vi "Main.vi"() -> ()   [LabVIEW 2017]
doc: "The myRIO Project template acquires acceleration data from the onboard accelerometer and displays the changes of acceleration values in a waveform chart."
uses:
  <vilib>/myRIO/Instrument Drivers/Onboard IO/I2C/typedefs/I2C User Configuration.ctl
  <vilib>/myRIO/Instrument Drivers/Onboard IO/I2C/typedefs/I2C Transfer Rate.ctl
  <vilib>/myRIO/Instrument Drivers/Onboard IO/I2C/typedefs/I2C Reference.ctl
  <vilib>/myRIO/Common/Instrument Driver Framework/Utilities/typedefs/myRIO Generic Hardware Reference.ctl
  <vilib>/myRIO/Common/Instrument Driver Framework/Utilities/typedefs/Hardware Version Enum.ctl
  <vilib>/myRIO/Common/Instrument Driver Framework/Utilities/typedefs/myRIO v1.0 Reference.ctl
  <vilib>/myRIO/Common/Instrument Driver Framework/Utilities/typedefs/Generic FPGA Reference.ctl
  <vilib>/myRIO/Common/Instrument Driver Framework/myRIO v1.0/I2C/typedefs/I2C Channels Enum.ctl
  <vilib>/myRIO/Instrument Drivers/Onboard IO/I2C/typedefs/I2C Configuration.ctl
  <vilib>/userdefined/High Color/nirio_resource_hc.ctl
  <vilib>/myRIO/Common/Instrument Driver Framework/myRIO v1.0/I2C/vis/myRIO v1.1 Open I2C.vi
  <vilib>/myRIO/Common/Instrument Driver Framework/Utilities/vis/Validate Channels.vi
  <vilib>/myRIO/Common/Instrument Driver Framework/myRIO v1.0/I2C/vis/myRIO v1.0 Reserve I2C.vi
  <vilib>/myRIO/Common/Instrument Driver Framework/myRIO v1.0/UART/vis/myRIO v1.0 Close UART.vi
  <vilib>/myRIO/Common/Instrument Driver Framework/myRIO v1.0/I2C/vis/myRIO v1.0 Build MUX Configuration I2C.vi
  <vilib>/myRIO/Common/Instrument Driver Framework/myRIO v1.0/Resource Manager/vis/myRIO v1.0 Reserve Channel List.vi
  <vilib>/myRIO/Common/Instrument Driver Framework/myRIO v1.0/Resource Manager/vis/myRIO v1.0 Create Configuration List.vi
  <vilib>/myRIO/Common/Instrument Driver Framework/myRIO v1.0/Resource Manager/vis/myRIO v1.0 Reserve Channel.vi
  <vilib>/myRIO/Common/Instrument Driver Framework/myRIO v1.0/Resource Manager/vis/myRIO v1.0 Unreserve Channel.vi
  <vilib>/myRIO/Common/Instrument Driver Framework/myRIO v1.0/Resource Manager/vis/myRIO v1.0 Build Mutex Name.vi
  <vilib>/Utility/VariantDataType/GetNumericInfo.vi
  <vilib>/Utility/error.llb/Error Cluster From Error Code.vi
  <vilib>/myRIO/Common/Instrument Driver Framework/myRIO v1.0/myRIO v1.1 Open.vi
  <vilib>/myRIO/Common/Instrument Driver Framework/Utilities/vis/IO Manager.vi
  <vilib>/myRIO/Common/Instrument Driver Framework/Utilities/vis/Configuration Manager.vi
  <vilib>/myRIO/Common/Instrument Driver Framework/myRIO v1.0/Resource Manager/vis/myRIO v1.0 Configure IO.vi
  <vilib>/myRIO/Common/Instrument Driver Framework/myRIO v1.0/myRIO v1.0 Close.vi
  <vilib>/myRIO/Common/Instrument Driver Framework/myRIO v1.0/I2C/vis/myRIO v1.0 Configure I2C.vi
  <vilib>/myRIO/Common/Instrument Driver Framework/myRIO v1.0/I2C/vis/myRIO v1.0 Write I2C.vi
  <vilib>/myRIO/Common/Instrument Driver Framework/myRIO v1.0/I2C/vis/myRIO v1.0 Read I2C.vi
  <vilib>/myRIO/Common/Instrument Driver Framework/Utilities/vis/FPGA Ref Manager.vi
  <vilib>/myRIO/Common/Instrument Driver Framework/myRIO v1.0/myRIO v1.0 Reset FPGA.vi
  <vilib>/myRIO/Common/Instrument Driver Framework/myRIO v1.0/IRQ/vis/myRIO v1.0 IRQ Info FGV.vi
  <vilib>/myRIO/Common/Instrument Driver Framework/myRIO v1.0/IRQ/vis/myRIO v1.0 Timer IRQ Info FGV.vi
  <vilib>/myRIO/Common/Instrument Driver Framework/myRIO v1.0/IRQ/vis/myRIO v1.0 ISR Agent.vi
  <vilib>/myRIO/Instrument Drivers/Onboard IO/I2C/vis/myRIO I2C Open.xnode
  <vilib>/myRIO/Instrument Drivers/Utilities/Utilities.lvlib
  <vilib>/myRIO/Instrument Drivers/Onboard IO/I2C/I2C.lvlib
  <vilib>/ptbypt/NI_PtbyPt.lvlib
panel:
  out "AC estimate (Vrms)":dbl format="%0.2f"
  out "DC estimate (V)":dbl format="%0.2f"
  out "l":u8
  out "h":u8
  out "Numeric Control":u16
  out "error out":errorcluster
  in  "Stop":bool
  # "Overview: The myRIO Project template acquires acceleration data from the onboard accelerometer and displays the changes of acceleration values in a waveform chart.\nInstructions:\n1. Check the myRIO target IP address in the project and make sure the target IP address is correct. \n2. Run this VI."
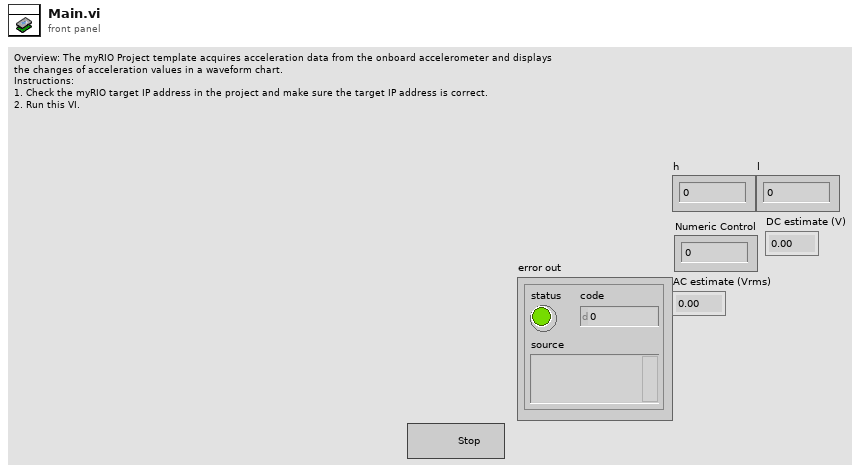
[diagram p1: front panel]
types:
  T1 = typedef "I2C.lvlib/I2C User Configuration.ctl" = cluster{"I2C Transfer Rate":T2}
  T2 = typedef "I2C.lvlib/I2C Transfer Rate.ctl" = enum16{"Standard mode (100 kbps)", "Fast mode (400 kbps)"}
  T3 = typedef "nirio_resource_hc.ctl" = tag
  T4 = typedef "Hardware Version Enum.ctl" = enum16{"Unknown", "myRIO-1900", "myRIO-1950", "roboRIO", "NI ELVIS RIO CM"}
  T5 = typedef "I2C.lvlib/I2C Reference.ctl" = cluster{"myRIO Reference":T6, "I2C Channels Enum":T9, "I2C Configuration":T10}
  T6 = typedef "myRIO Generic Hardware Reference.ctl" = cluster{"myRIO Model":T4, "myRIO Hardware Reference":T7}
  T7 = typedef "myRIO v1.0 Reference.ctl" = cluster{"Generic FPGA Reference":T8, "Allow multiple opens":bool}
  T8 = typedef "Generic FPGA Reference.ctl" = refnum<k20>
  T9 = typedef "I2C Channels Enum.ctl" = enum16{"Not Connected", "A/I2C", "B/I2C", "I2C/I2C"}
  T10 = typedef "I2C.lvlib/I2C Configuration.ctl" = cluster{"I2C Transfer Rate":T2}
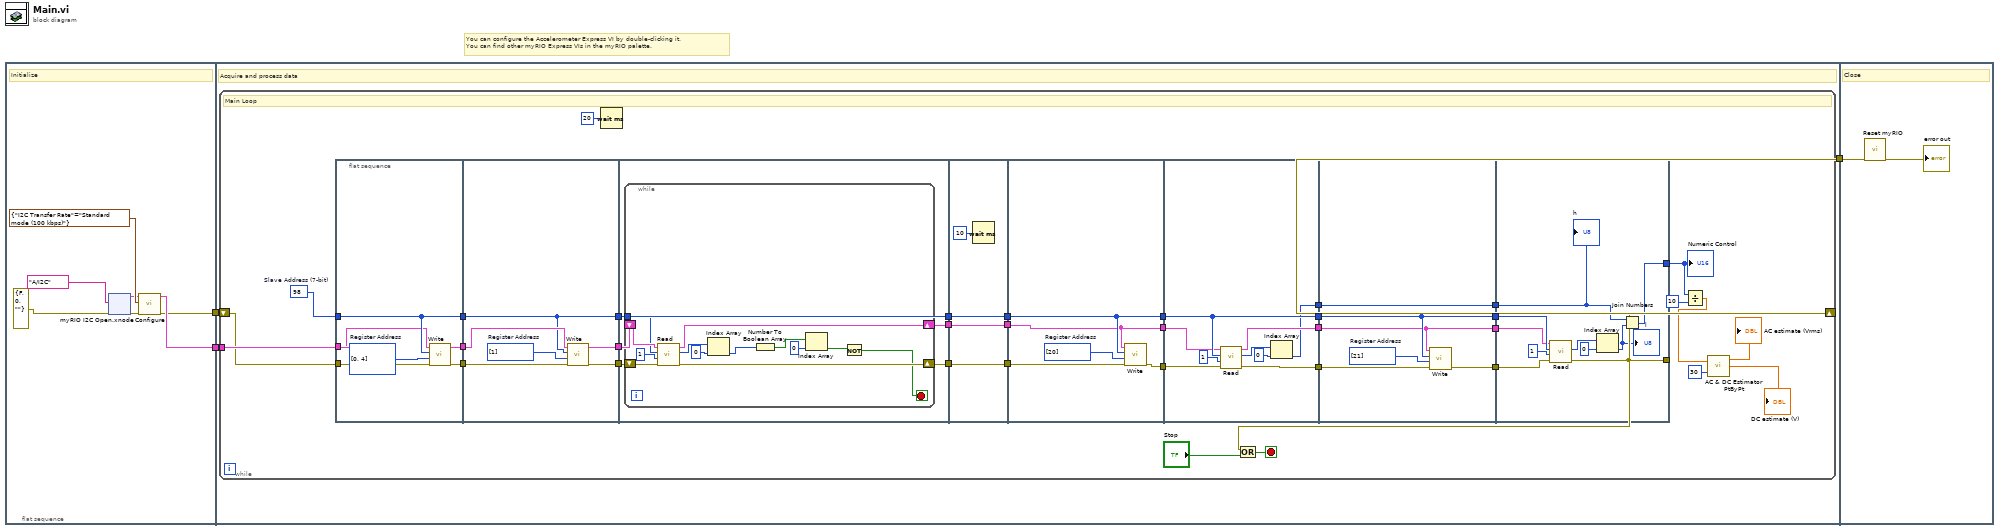
[diagram p0: block diagram]
diagram:
  # "You can configure the Accelerometer Express VI by double-clicking it.\nYou can find other myRIO Express VIs in the myRIO palette."
  n1 = flat-sequence {
    tunnel: [w5] -> w2
    tunnel: [w4] -> w1
    tunnel: [w28] -> w3
    tunnel: w2 -> [w27]
    tunnel: w1 -> [w29]
    tunnel: w3 -> [w131]
    frame #0 {
      # "Initialize"
      n2 = xnode "myRIO I2C Open.xnode"("error in (no error)"=errorcluster {"status"=FALSE, "code"=0, "source"=""}, "Channel Name"=tag "A/I2C") -> ("error out"=w7:errorcluster, "I2C Ref Out"=w8:T5)  [unwired: 1 in]
      n3 = call <vilib>:"Configure.vi"("error in (no error)"=w7, "I2C User Configuration"=T1 {"I2C Transfer Rate"=enum."Standard mode (100 kbps)"}, "I2C Ref In"=w8) -> ("error out"=w4:errorcluster, "I2C Ref Out"=w5:T5)  [unwired: 7 in]
    }
    frame #1 {
      # "Acquire and process data"
      n4 = while {
        shift-right: [w42] -> w28
        shift-left: w29 -> [w60]
        tunnel: w27 -> [w61]
        stop <- w64 stop-if-true
        w62 = u8 98  # Slave Address (7-bit)
        # "Main Loop"
        n5 = flat-sequence {
          tunnel: [w71] -> w59
          tunnel: [w70] -> w57
          tunnel: w62 -> [w68]
          tunnel: [w68] -> w55
          tunnel: w61 -> [w67]
          tunnel: w60 -> [w66]
          tunnel: w59 -> [w74]
          tunnel: [w73] -> w58
          tunnel: w57 -> [w75]
          tunnel: [w76] -> w56
          tunnel: w55 -> [w72]
          tunnel: [w72] -> w54
          tunnel: w58 -> [w82]
          tunnel: w56 -> [w81]
          tunnel: w54 -> [w78]
          tunnel: [w80] -> w41
          tunnel: [w79] -> w39
          tunnel: [w78] -> w37
          tunnel: w41 -> [w99]
          tunnel: [w99] -> w40
          tunnel: w39 -> [w98]
          tunnel: [w98] -> w38
          tunnel: w37 -> [w97]
          tunnel: [w97] -> w36
          tunnel: w40 -> [w100]
          tunnel: w38 -> [w103]
          tunnel: w36 -> [w101]
          tunnel: [w102] -> w53
          tunnel: [w101] -> w49
          tunnel: [w100] -> w45
          tunnel: w53 -> [w110]
          tunnel: [w109] -> w52
          tunnel: [w108] -> w50
          tunnel: w49 -> [w107]
          tunnel: [w107] -> w48
          tunnel: w45 -> [w106]
          tunnel: [w105] -> w44
          tunnel: w52 -> [w118]
          tunnel: [w117] -> w51
          tunnel: w50 -> [w115]
          tunnel: w48 -> [w116]
          tunnel: [w116] -> w47
          tunnel: [w115] -> w46
          tunnel: w44 -> [w114]
          tunnel: [w114] -> w43
          tunnel: w51 -> [w126]
          tunnel: w47 -> [w125]
          tunnel: w46 -> [w124]
          tunnel: w43 -> [w120]
          tunnel: [w123] -> w42
          tunnel: [w122] -> w35
          frame #0 {
            w69 = u8[] [0, 4]  # Register Address
            n6 = call <vilib>:"Write.vi"("error in (no error)"=w66, "Bytes to Write"=w69, "Slave Address (7-bit)"=w68, "I2C Ref In"=w67) -> ("error out"=w70:errorcluster, "I2C Ref Out"=w71:T5)  [unwired: 6 in]
          }
          frame #1 {
            w77 = u8[] [1]  # Register Address
            n7 = call <vilib>:"Write.vi"("error in (no error)"=w75, "Bytes to Write"=w77, "Slave Address (7-bit)"=w72, "I2C Ref In"=w74) -> ("error out"=w76:errorcluster, "I2C Ref Out"=w73:T5)  [unwired: 6 in]
          }
          frame #2 {
            n8 = while {
              tunnel: w78 -> [w88]
              shift-right: [w90] -> w80
              shift-left: w82 -> [w94]
              shift-right: [w89] -> w79
              shift-left: w81 -> [w91]
              stop <- w83 stop-if-true
              n9 = call <vilib>:"Read.vi"("error in (no error)"=w91, "Byte Count"=u32 1, "Slave Address (7-bit)"=w88, "I2C Ref In"=w94) -> ("error out"=w89:errorcluster, "Bytes Read"=w93:u8[], "I2C Ref Out"=w90:T5)  [unwired: 4 in]
              n10 = Index Array(array=w93, index=0) -> (element=w87:u8)
              n11 = Number To Boolean Array(number=w87) -> (Boolean array=w86:bool[])
              n12 = Index Array(array=w86, index=0) -> (element=w84:bool)
              n13 = Not(x=w84) -> (.not. x?=w83:bool)
            }
          }
          frame #3 {
            n14 = Wait (ms)(milliseconds to wait=u32 10) -> ()  [unwired: 1 out]
          }
          frame #4 {
            w104 = u8[] [20]  # Register Address
            n15 = call <vilib>:"Write.vi"("error in (no error)"=w103, "Bytes to Write"=w104, "Slave Address (7-bit)"=w101, "I2C Ref In"=w100) -> ("error out"=w102:errorcluster)  [unwired: 6 in, 1 out]
          }
          frame #5 {
            n16 = call <vilib>:"Read.vi"("error in (no error)"=w110, "Byte Count"=u32 1, "Slave Address (7-bit)"=w107, "I2C Ref In"=w106) -> ("error out"=w109:errorcluster, "Bytes Read"=w112:u8[], "I2C Ref Out"=w108:T5)  [unwired: 4 in]
            n17 = Index Array(array=w112, index=0) -> (element=w105:u8)
          }
          frame #6 {
            w119 = u8[] [21]  # Register Address
            n18 = call <vilib>:"Write.vi"("error in (no error)"=w118, "Bytes to Write"=w119, "Slave Address (7-bit)"=w116, "I2C Ref In"=w115) -> ("error out"=w117:errorcluster)  [unwired: 6 in, 1 out]
          }
          frame #7 {
            n19 = call <vilib>:"Read.vi"("error in (no error)"=w126, "Byte Count"=u32 1, "Slave Address (7-bit)"=w125, "I2C Ref In"=w124) -> ("error out"=w123:errorcluster, "Bytes Read"=w128:u8[])  [unwired: 4 in, 1 out]
            n20 = Index Array(array=w128, index=0) -> (element=w121:u8)
            "l" <- w121
            n21 = Join Numbers(hi=w120, lo=w121) -> ((hi.lo)=w122:u16)
            "h" <- w120
          }
        }
        n22 = Wait (ms)(milliseconds to wait=u32 20) -> ()  [unwired: 1 out]
        n23 = Or(x=w42, y="Stop") -> (x .or. y?=w64:bool)
        n24 = Divide(x=w35, y=u16 10) -> (x/y=w33:dbl)
        n25 = call <vilib>:"AC & DC Estimator PtByPt.vi"("signal"=w33, "sample length"=30) -> ("AC estimate (Vrms)"=→"AC estimate (Vrms)":dbl, "DC estimate (V)"=→"DC estimate (V)":dbl)  [unwired: 1 in, 1 out]
        "Numeric Control" <- w35
      }
    }
    frame #2 {
      # "Close"
      n26 = call <vilib>:"Reset myRIO.vi"("error in (no error)"=w131) -> ("error out"=→"error out":errorcluster)  [unwired: 10 in]
    }
  }
